vi "fo_SendFileExe.vi"(8 "error in (no error)":errorcluster, 10 "ServerInfo":T1={"port"=104, "AEtitle"="ME", "host"="127.0.0.1", "remoteAE"="STORESCP"}, 11 "File":string) -> (0 "error out":errorcluster)   [LabVIEW 2013, in "main.lvlib"]
uses:
  main.lvlib
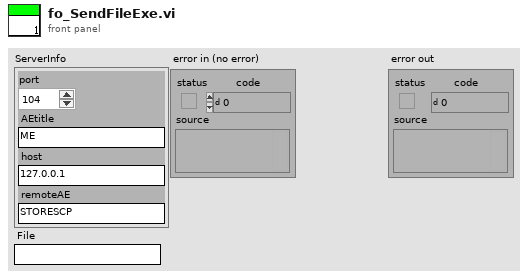
[diagram p1: front panel]
types:
  T1 = cluster{"port":i32, "AEtitle":string, "host":string, "remoteAE":string}
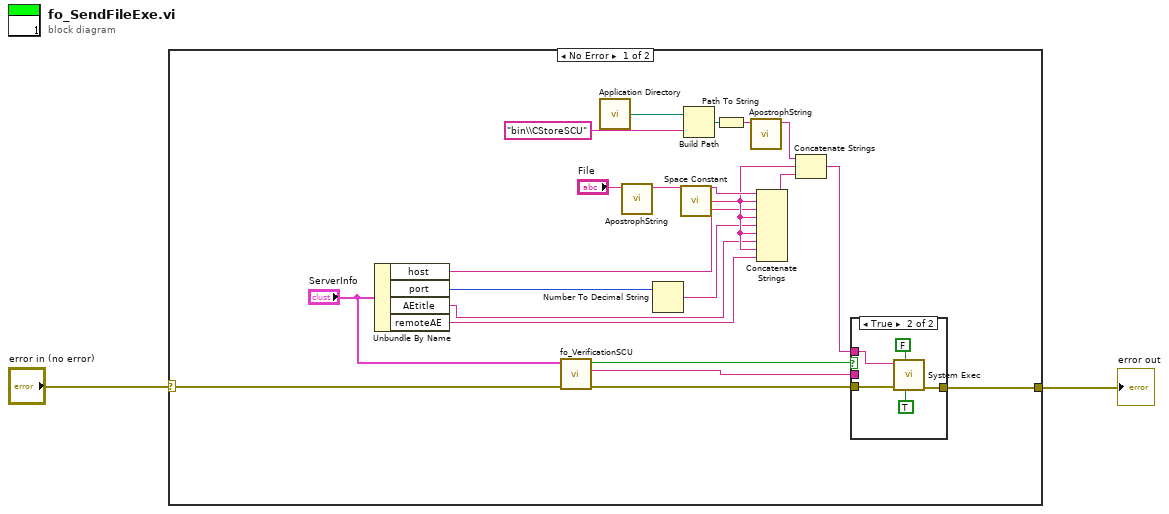
[diagram p0: block diagram]
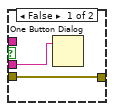
[diagram p2: hidden frame]
diagram:
  n1 = case shown="No Error" "error in (no error)" {
    selector: "error in (no error)" -> [w4 w31]
    tunnel: [w3 w31] -> w1
    frame No Error {
      n2 = Unbundle By Name("ServerInfo") -> ("host"=w10:string, "port"=w9:i32, "AEtitle"=w12:string, "remoteAE"=w11:string)
      n3 = call "fo_VerificationSCU.vi"("error in (no error)"=w4, "ServerInfo"="ServerInfo") -> ("error out"=w7:errorcluster, "status"=w5:string, "Succes?"=w6:bool)  [unwired: 7 in]
      n4 = call <vilib>:"Application Directory.vi"() -> ("Application Directory"=w22:path)
      n5 = call "ApostrophString.vi"("String in"="File") -> ("String out"=w23:string)  [unwired: 10 in]
      n6 = Number To Decimal String(number=w9) -> (decimal integer string=w13:string)  [unwired: 1 in]
      n7 = call <vilib>:"Space Constant.vi"() -> ("String"=w14:string)
      n8 = Build Path(base path=w22, name or relative path="bin\\CStoreSCU") -> (appended path=w20:path)
      n9 = Path To String(path=w20) -> (string=w19:string)
      n10 = call "ApostrophString.vi"("String in"=w19) -> ("String out"=w17:string)  [unwired: 10 in]
      n11 = Concatenate Strings(w23, w14, w10, w14, w13, w14, w12, w14, w11) -> (w18:string)
      n12 = Concatenate Strings(w17, w14, w18) -> (w16:string)
      n13 = case shown="True" w6 {
        tunnel: w16 -> [_ w28]
        tunnel: [w25 w29] -> w3
        tunnel: w7 -> [w25 w26]
        tunnel: w5 -> [w24 _]
        frame False {
          n14 = One Button Dialog(message=w24) -> ()  [unwired: 1 in, 1 out]
        }
        frame True {
          n15 = call <vilib>:"System Exec.vi"("run minimized? (F)"=TRUE, "wait until completion? (T)"=FALSE, "error in (no error)"=w26, "command line"=w28) -> ("error out"=w29:errorcluster)  [unwired: 4 in, 3 out]
        }
      }
    }
    frame Error {
    }
  }
  "error out" <- w1
